vi "modify_cell_approach.vi"(5 "approach above cell (steps)":i32, 6 "approach type":T3=enum."vertical abs", 7 "which manipulator":T2(ring), 8 "abs or rel park location (z only) (px)":i32[](array[numeric]), 9 "transform cluster + actuator":T4, 10 "current positions":T1, 11 "cell location (steps, pipette coord system)":dbl[](array[numeric])) -> (0 "distToDescend (steps)":i32, 2 "approach cell location (px)":dbl[](array[numeric]), 3 "approach cell location (steps, pipette coord system)":dbl[](array[numeric]))   [LabVIEW 2015]
uses:
  controls/approach_type.ctl
  pipette cleaning/pressure box/cleaning_soft/controls/actuator_type.ctl
  pipette cleaning/pressure box/cleaning_soft/controls/actuator_cluster.ctl
  transform_properties_actuators.ctl
  controls/transform_cluster_actuator.ctl
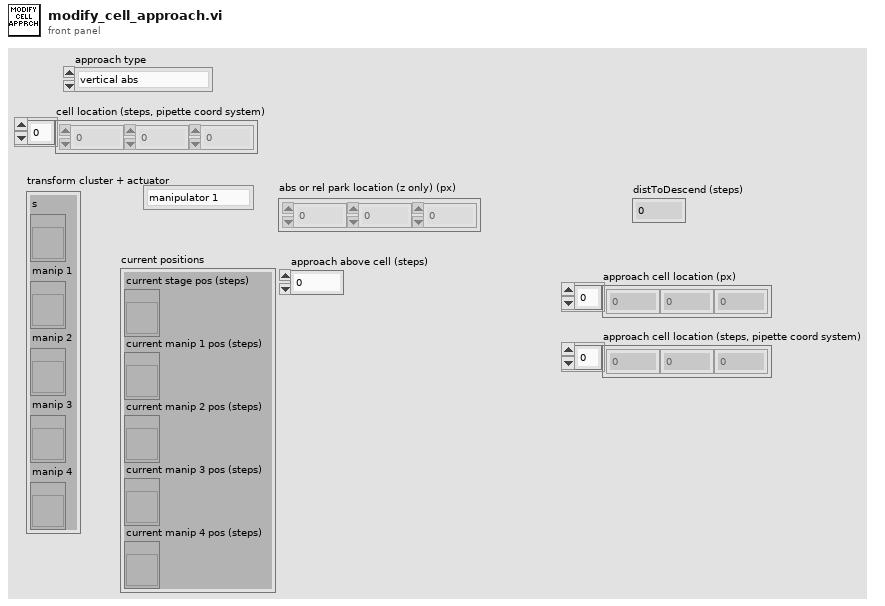
[diagram p1: front panel]
types:
  T1 = cluster{"current stage pos (steps)":refnum<vi>, "current manip 1 pos (steps)":refnum<vi>, "current manip 2 pos (steps)":refnum<vi>, "current manip 3 pos (steps)":refnum<vi>, "current manip 4 pos (steps)":refnum<vi>}
  T2 = enum16{"manipulator 1", "manipulator 2", "manipulator 3", "manipulator 4"}
  T3 = typedef "approach_type.ctl" = enum16{"right to cell", "vertical abs", "approach", "vertical rel", "approach above"}
  T4 = typedef "transform_cluster_actuator.ctl" = cluster{"s":refnum<vi>, "manip 1":refnum<vi>, "manip 2":refnum<vi>, "manip 3":refnum<vi>, "manip 4":refnum<vi>}
  T5 = typedef "transform_properties_actuators.ctl" = cluster{"theta (deg)":dbl, "X sc factor (px/step)":dbl, "Y sc factor (px/step)":dbl, "zero loc (x,y,z)":dbl[], "flip y?":bool, "flip x?":bool, "gamma (deg)":dbl, "flip z?":bool, "Z sc factor (px/step)":dbl, "actuator":T6, "safe space (steps)":i32[]}
  T6 = typedef "actuator_cluster.ctl" = cluster{"Actuator COM":refnum<visa-resource-name>, "Actuator type":T7}
  T7 = typedef "actuator_type.ctl" = enum16{"Scientifica", "Sutter", "Demo", "Off"}
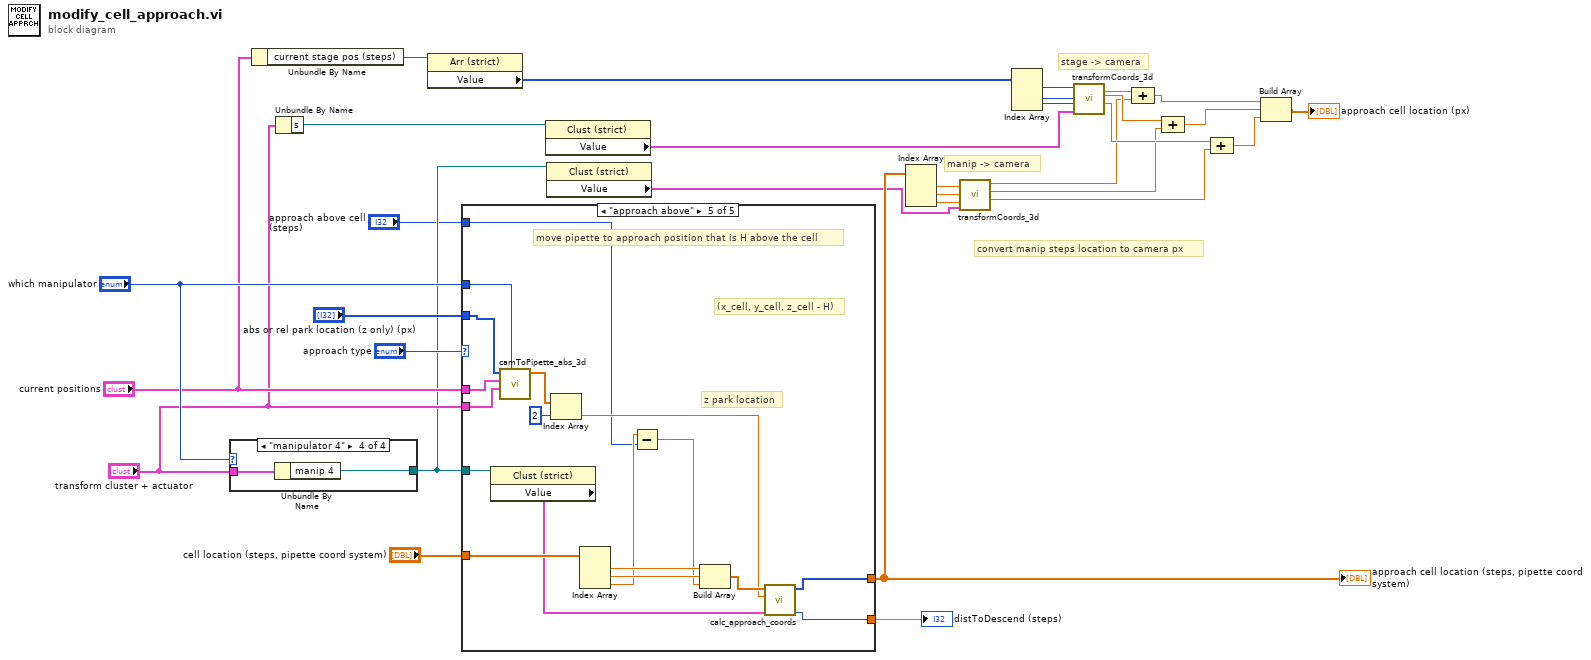
[diagram p0: block diagram]
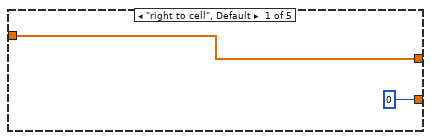
[diagram p2: hidden frame]
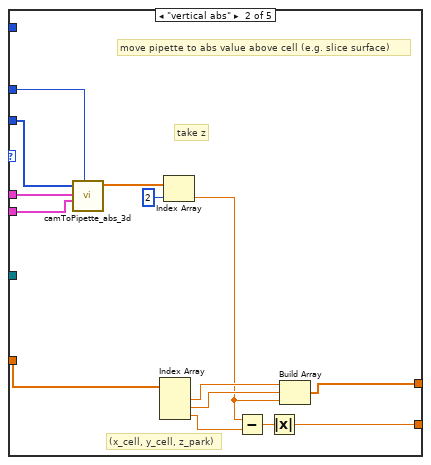
[diagram p3: hidden frame]
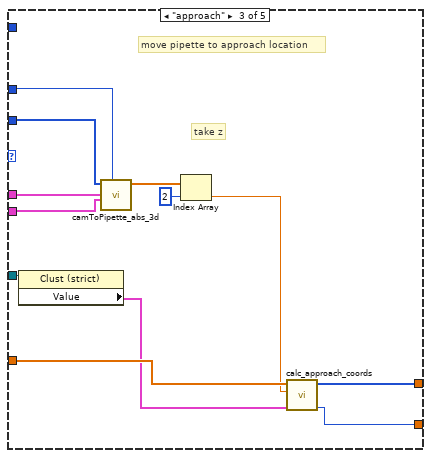
[diagram p4: hidden frame]
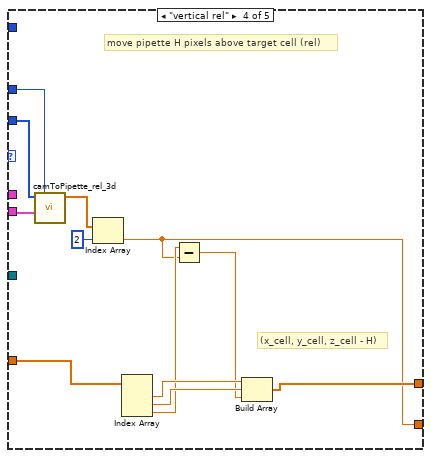
[diagram p5: hidden frame]
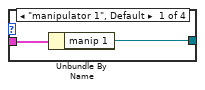
[diagram p6: hidden frame]
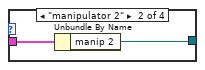
[diagram p7: hidden frame]
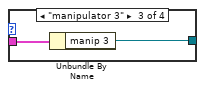
[diagram p8: hidden frame]
diagram:
  # "manip -> camera"
  # "stage -> camera"
  # "convert manip steps location to camera px"
  n1 = case shown="\"manipulator 4\"" "which manipulator" {
    tunnel: "transform cluster + actuator" -> [w33 w35 w37 w39]
    tunnel: [w32 w34 w36 w38] -> w11
    frame "manipulator 1", Default {
      n2 = Unbundle By Name(w33) -> ("manip 1"=w32:refnum<vi>)
    }
    frame "manipulator 2" {
      n3 = Unbundle By Name(w35) -> ("manip 2"=w34:refnum<vi>)
    }
    frame "manipulator 3" {
      n4 = Unbundle By Name(w37) -> ("manip 3"=w36:refnum<vi>)
    }
    frame "manipulator 4" {
      n5 = Unbundle By Name(w39) -> ("manip 4"=w38:refnum<vi>)
    }
  }
  n6 = Unbundle By Name("current positions") -> ("current stage pos (steps)"=w24:refnum<vi>)
  n7 = Unbundle By Name("transform cluster + actuator") -> ("s"=w21:refnum<vi>)
  n8 = property class="Arr (strict)"(reference=w24) -> ("Value"=w23:i32[])  [unwired: 1 in, 2 out]
  n9 = case shown="\"approach above\"" "approach type" {
    tunnel: "cell location (steps, pipette coord system)" -> [w41 w55 w65 w76 w91]
    tunnel: [w41 w51 w63 w74 w85] -> w26
    tunnel: w11 -> [_ _ w66 _ w90]
    tunnel: "which manipulator" -> [_ w46 w60 w69 w84]
    tunnel: "abs or rel park location (z only) (px)" -> [_ w45 w59 w70 w80]
    tunnel: "current positions" -> [_ w43 w57 _ w82]
    tunnel: "transform cluster + actuator" -> [_ w44 w61 w71 w81]
    tunnel: [0 ("distToDescend") w47 w62 w72 w86] -> w27
    tunnel: "approach above cell (steps)" -> [_ _ _ _ w87]
    frame "right to cell", Default {
    }
    frame "vertical abs" {
      # "move pipette to abs value above cell (e.g. slice surface)"
      # "(x_cell, y_cell, z_park)"
      # "take z"
      n10 = call "camToPipette_abs_3d.vi"("which manipulator"=w46, "transform cluster + actuator"=w44, "current positions"=w43, "abs pixel location"=w45) -> ("pipette location (steps)"=w42:dbl[])  [unwired: 7 in]
      n11 = Index Array(array=w55) -> (element #1=w54:dbl, element #2=w53:dbl, element #3=w49:dbl)  [unwired: 3 in]
      n12 = Index Array(array=w42, index=2) -> (element=w50:dbl)
      n13 = Subtract(x=w50, y=w49) -> (x-y=w48:dbl)
      n14 = Absolute Value(x=w48) -> (abs(x)=w47:dbl)
      n15 = Build Array(w54, w53, w50) -> (w51:dbl[])
    }
    frame "approach" {
      # "move pipette to approach location"
      # "take z"
      n16 = property class="Clust (strict)"(reference=w66) -> ("Value"=w56:T5)  [unwired: 1 in, 2 out]
      n17 = call "camToPipette_abs_3d.vi"("which manipulator"=w60, "transform cluster + actuator"=w61, "current positions"=w57, "abs pixel location"=w59) -> ("pipette location (steps)"=w58:dbl[])  [unwired: 7 in]
      n18 = Index Array(array=w58, index=2) -> (element=w64:dbl)
      n19 = call "calc_approach_coords.vi"("manip transform"=w56, "Z_topP"=w64, "cell location (steps, pipette coord system)"=w65) -> ("distToDescend"=w62:i32, "(x,y,z)_pP_TOPOFSLICE"=w63:i32[])  [unwired: 7 in]
    }
    frame "vertical rel" {
      # "(x_cell, y_cell, z_cell - H)"
      # "move pipette H pixels above target cell (rel)"
      n20 = call "camToPipette_rel_3d.vi"("which manipulator"=w69, "transform cluster + actuator"=w71, "rel cam (px)"=w70) -> ("rel pipette (steps)"=w68:dbl[])  [unwired: 8 in]
      n21 = Index Array(array=w68, index=2) -> (element=w72:dbl)
      n22 = Index Array(array=w76) -> (element #1=w78:dbl, element #2=w77:dbl, element #3=w73:dbl)  [unwired: 3 in]
      n23 = Subtract(x=w73, y=w72) -> (x-y=w75:dbl)
      n24 = Build Array(w78, w77, w75) -> (w74:dbl[])
    }
    frame "approach above" {
      # "z park location"
      # "move pipette to approach position that is H above the cell"
      # "(x_cell, y_cell, z_cell - H)"
      n25 = property class="Clust (strict)"(reference=w90) -> ("Value"=w89:T5)  [unwired: 1 in, 2 out]
      n26 = call "camToPipette_abs_3d.vi"("which manipulator"=w84, "transform cluster + actuator"=w81, "current positions"=w82, "abs pixel location"=w80) -> ("pipette location (steps)"=w83:dbl[])  [unwired: 7 in]
      n27 = Index Array(array=w83, index=2) -> (element=w88:dbl)
      n28 = Index Array(array=w91) -> (element #1=w96:dbl, element #2=w95:dbl, element #3=w93:dbl)  [unwired: 3 in]
      n29 = Subtract(x=w93, y=w87) -> (x-y=w94:dbl)
      n30 = Build Array(w96, w95, w94) -> (w92:dbl[])
      n31 = call "calc_approach_coords.vi"("manip transform"=w89, "Z_topP"=w88, "cell location (steps, pipette coord system)"=w92) -> ("distToDescend"=w86:i32, "(x,y,z)_pP_TOPOFSLICE"=w85:i32[])  [unwired: 7 in]
    }
  }
  "approach cell location (steps, pipette coord system)" <- w26
  "distToDescend (steps)" <- w27
  n32 = property class="Clust (strict)"(reference=w21) -> ("Value"=w20:T5)  [unwired: 1 in, 2 out]
  n33 = property class="Clust (strict)"(reference=w11) -> ("Value"=w10:T5)  [unwired: 1 in, 2 out]
  n34 = Index Array(array=w26) -> (element #1=w14:dbl, element #2=w13:dbl, element #3=w12:dbl)  [unwired: 3 in]
  n35 = call "transformCoords_3d.vi"("transform properties"=w10, "z"=w12, "y"=w13, "x"=w14) -> ("z out"=w6:dbl, "y out"=w7:dbl, "x out"=w8:dbl)  [unwired: 5 in]
  n36 = Index Array(array=w23) -> (element #1=w19:i32, element #2=w18:i32, element #3=w17:i32)  [unwired: 3 in]
  n37 = call "transformCoords_3d.vi"("transform properties"=w20, "z"=w17, "y"=w18, "x"=w19) -> ("z out"=w9:dbl, "y out"=w15:dbl, "x out"=w16:dbl)  [unwired: 5 in]
  n38 = Compound Arithmetic op=ADD(w16, w8) -> (w5:dbl)
  n39 = Compound Arithmetic op=ADD(w15, w7) -> (w4:dbl)
  n40 = Compound Arithmetic op=ADD(w9, w6) -> (w3:dbl)
  n41 = Build Array(w5, w4, w3) -> (→"approach cell location (px)":dbl[])
